vi "XLP80_Action_Testmode_A_Write_DCDC.vi"(7 "CAN Write Items Testmode_A":T1=enum."LV_A_71_Voltage_In_Set", 8 "err in":errorcluster, 11 "DCDC Write":dbl=1.0) -> (0 "err out":errorcluster)   [LabVIEW 2021]
uses:
  XLP80_FGlob/1886_FGlob_TDefEnumCANWriteItems.ctl
  XLP80_FGlob/1886_FGlob_TDefs_Enum_FGlobItems.ctl
  XLP80_Globals/XLP80_Globals_Referenzen.vi
  XLP80_Globals/XLP80_CAN_Globals.vi
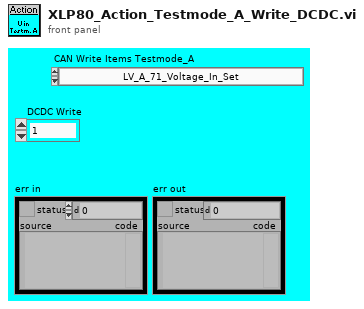
[diagram p1: front panel]
types:
  T1 = typedef "1886_FGlob_TDefEnumCANWriteItems.ctl" = enum16{"LV_Testmode_Select", "LV_A_71_Current_Out_Set", "LV_A_71_Voltage_In_Set", "LV_A_71_Voltage_Out_Set", "LV_H_51_STK_CellVoltages_Enable", "S80_BP_s_Taster_Start_Status"}
  T2 = typedef "1886_FGlob_TDefs_Enum_FGlobItems.ctl" = enum16{"Put one", "Put all", "Recall one", "Recall all"}
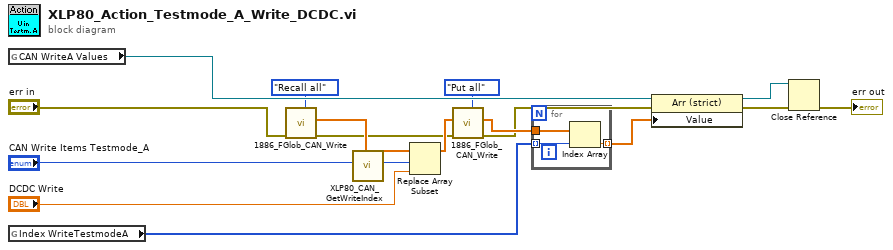
[diagram p0: block diagram]
diagram:
  n1 = global read "XLP80_Globals_Referenzen.vi" "CAN WriteA Values"() -> (w15:refnum<vi>)
  n2 = global read "XLP80_CAN_Globals.vi" "Index WriteTestmodeA"() -> (w17:i32[])
  n3 = call "1886_FGlob_CAN_Write.vi"("Function (Recall One)"=1886_FGlob_TDefs_Enum_FGlobItems."Recall all", "err in"="err in") -> ("err out"=w8:errorcluster, "AO Values OUT"=w10:dbl[])  [unwired: 7 in, 1 out]
  n4 = call "XLP80_CAN_GetWriteIndex.vi"("CAN Write Items"="CAN Write Items Testmode_A") -> ("Index"=w13:i32)  [unwired: 10 in]
  n5 = Replace Array Subset(array=w10, new element="DCDC Write", index=w13) -> (w9:dbl[])
  n6 = call "1886_FGlob_CAN_Write.vi"("Function (Recall One)"=1886_FGlob_TDefs_Enum_FGlobItems."Put all", "err in"=w8, "AO Values IN"=w9) -> ("err out"=w5:errorcluster, "AO Values OUT"=w7:dbl[])  [unwired: 6 in, 1 out]
  n7 = for {
    tunnel: w17 -> [w19] mode=indexing
    tunnel: w7 -> [w20]
    tunnel: [w18] -> w6 mode=indexing
    n8 = Index Array(array=w20, index=w19) -> (element=w18:dbl)
  }
  n9 = property class="Arr (strict)"(reference=w15, error in=w5, "Value"=w6) -> (reference out=w3:refnum<vi>, error out=w4:errorcluster)
  n10 = Close Reference(reference=w3, error in (no error)=w4) -> (error out=→"err out":errorcluster)
